vi "Actor Core.vi"(8 "error in":errorcluster, 11 "User Interface in":refnum<class "User Interface.lvclass">) -> (0 "error out":errorcluster, 3 "Actor out":refnum<class "Actor.lvclass">)   [LabVIEW 2022 SP3, in "User Interface.lvlib" / "User Interface.lvclass"]
doc: "(<B>Filename</B>: Actor Framework.lvlib:Actor.lvclass:Actor Core.vi)\n\nReceives messages to the actor, reacts to them, and initiates any error handling that may shut the actor down.\n\nDescendant classes may override this VI to append parallel tasks for the actor to complete while it handles messages. Overrides use the Call Parent Class Method node."
uses:
  User Interface.lvclass
  User Interface.lvclass/User Interface.ctl
  <vilib>/ActorFramework/Actor/Actor.lvclass
  Controls/UI States.ctl
  User Interface.lvlib
  <vilib>/ActorFramework/Stop Msg/Stop Msg.lvclass
  C:/Program Files/National Instruments/LabVIEW 2022/vi.lib/ActorFramework/Actor/Actor.lvclass
  E:/image-harvest/User Interface/User Interface/User Interface.lvclass
panel:
  in  "Settings":bool
  in  "Stop":bool
  in  "Start":bool
  out "Progress Bar":u8(slide) scale=0.0..100.0
  in  "Listbox":i32(listbox)
  out "Image":T1(plugin-control)
  # "Start"
  # "Stop"
  # "Settings"
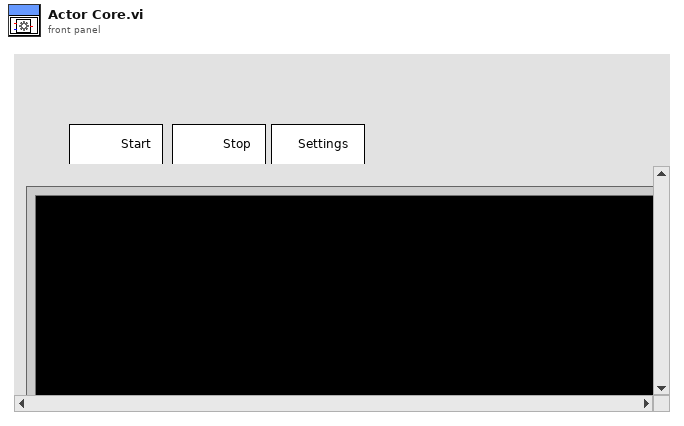
[diagram p1: front panel]
types:
  T1 = typedef "IMAQ Image.ctl" = refnum<image>
  T2 = typedef "User Interface.lvlib/UI States.ctl" = enum16{"Poll", "Initialize", "Start Acquisition", "Stop Acquisition", "Settings", "Error", "Exit"}
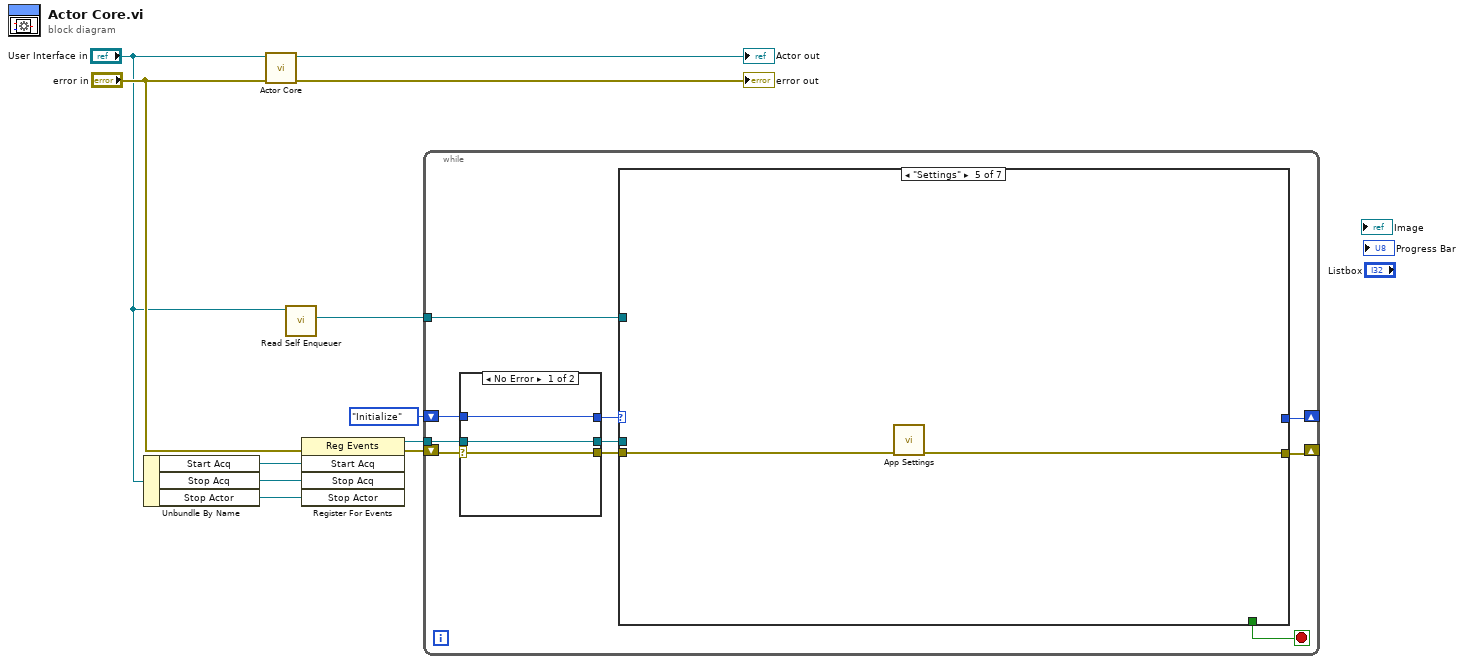
[diagram p0: block diagram]
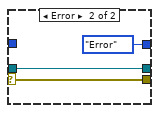
[diagram p2: hidden frame]
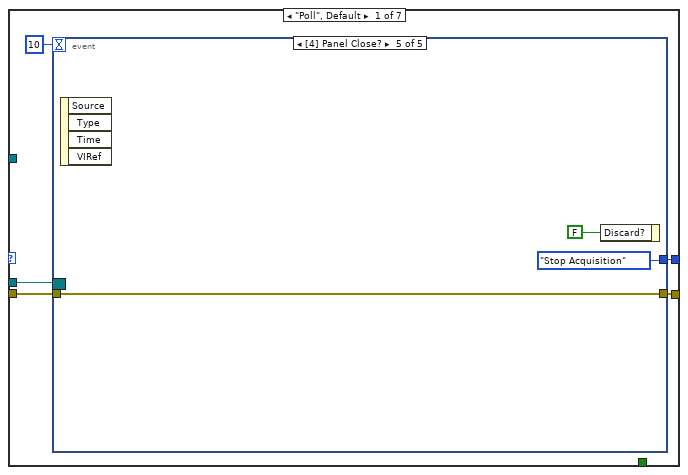
[diagram p3: hidden frame]
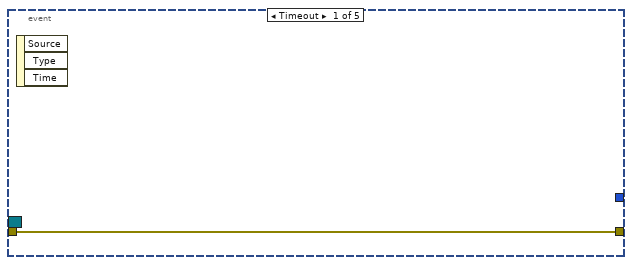
[diagram p4: hidden frame]
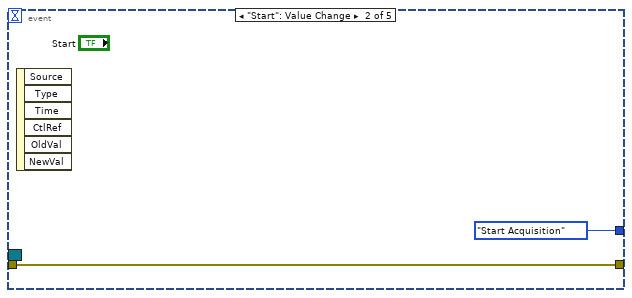
[diagram p5: hidden frame]
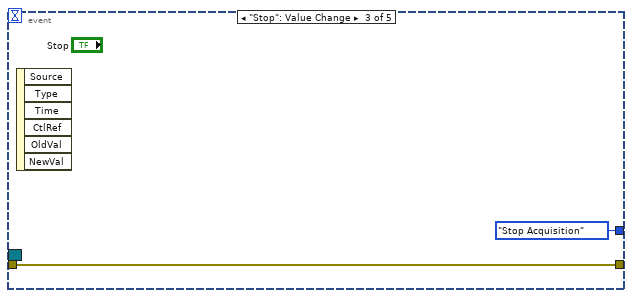
[diagram p6: hidden frame]
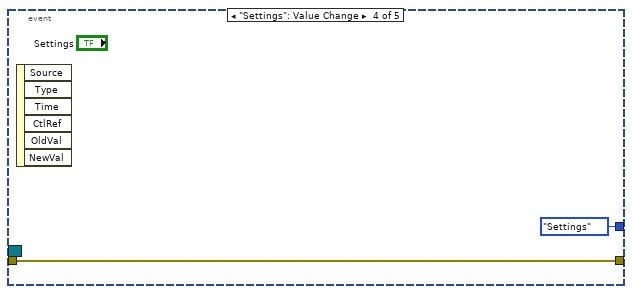
[diagram p7: hidden frame]
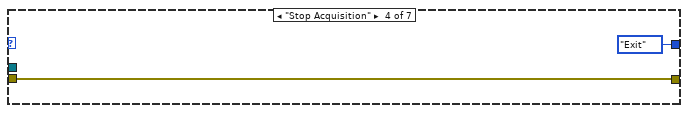
[diagram p10: hidden frame]
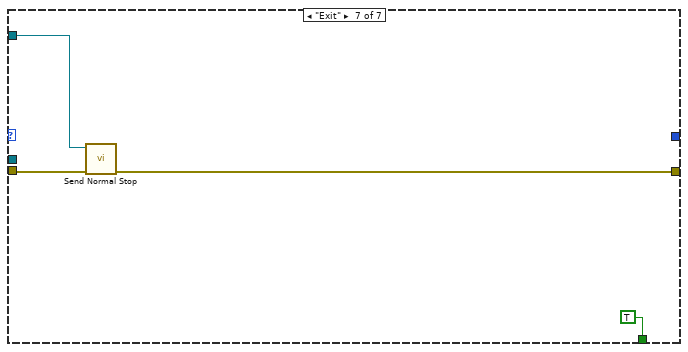
[diagram p12: hidden frame]
diagram:
  n1 = Unbundle By Name("User Interface in") -> ("Start Acq"=w8:refnum<user-event>, "Stop Acq"=w6:refnum<user-event>, "Stop Actor"=w7:refnum<user-event>)
  n2 = call-parent "Actor Core.vi"("error in"="error in", "Actor in"="User Interface in") -> ("error out"=→"error out":errorcluster, "Actor out"=→"Actor out":refnum<class "Actor.lvclass">)  [unwired: 8 in]
  n3 = call <vilib>:"Read Self Enqueuer.vi"("Actor"="User Interface in") -> ("Self Enqueuer"=w1:refnum<class "Message Enqueuer.lvclass">)  [unwired: 10 in]
  n4 = register-events(error in="error in", w8, w6, w7) -> (reference out=w4:refnum<event-registration>, error out=w3:errorcluster)  [unwired: 1 in]
  n5 = while {
    shift-right: [w21] -> _
    shift-left: UI_States."Initialize" -> [w18]
    tunnel: w4 -> [w17]
    shift-right: [w12] -> _
    shift-left: w3 -> [w20]
    tunnel: w1 -> [w13]
    stop <- w14 stop-if-true
    n6 = case shown="No Error" w20 {
      selector: w20 -> [w22 w26]
      tunnel: [w24 UI_States."Error"] -> w19
      tunnel: w18 -> [w24 _]
      tunnel: w17 -> [w23 w25]
      tunnel: [w23 w25] -> w16
      tunnel: [w22 w26] -> w15
      frame No Error {
      }
      frame Error {
      }
    }
    n7 = case shown="\"Settings\"" w19 {
      tunnel: w16 -> [w32 _ _ _ _ _ _]
      tunnel: [w31 _ _ UI_States."Exit" _ _ _] -> w21
      tunnel: w15 -> [w29 w43 w44 w46 w48 w49 w51]
      tunnel: [_ _ _ _ _ _ TRUE] -> w14
      tunnel: w13 -> [_ _ _ _ _ _ w52]
      tunnel: [w28 w43 w44 w46 w47 w49 w50] -> w12
      frame "Poll", Default {
        n8 = event shown="[4] Panel Close?" {
          selector: w32 -> [_ _ _ _ _]
          dyn-events: _ -> [_ _ _ _ _]
          timeout: 10 -> [_ _ _ _ _]
          tunnel: [_ UI_States."Start Acquisition" UI_States."Stop Acquisition" UI_States."Settings" UI_States."Stop Acquisition"] -> w31
          tunnel: w29 -> [w33 w34 w36 w38 w41]
          tunnel: [w33 w34 w36 w38 w41] -> w28
          event Timeout {
            n9 = event-data() -> ()  [unwired: 1 in, 3 out]
          }
          event "Start": Value Change {
            n10 = event-data() -> ()  [unwired: 1 in, 6 out]
          }
          event "Stop": Value Change {
            n11 = event-data() -> ()  [unwired: 1 in, 6 out]
          }
          event "Settings": Value Change {
            n12 = event-data() -> ()  [unwired: 1 in, 6 out]
          }
          event Panel Close? {
            n13 = event-data() -> ()  [unwired: 1 in, 4 out]
            n14 = event-data("Discard?"=FALSE) -> ()  [unwired: 1 in, 1 out]
          }
        }
      }
      frame "Initialize" {
      }
      frame "Start Acquisition" {
      }
      frame "Stop Acquisition" {
      }
      frame "Settings" {
        n15 = call "App Settings.vi"("Error in (no error)"=w48) -> ("Error out"=w47:errorcluster)  [unwired: 10 in]
      }
      frame "Error" {
      }
      frame "Exit" {
        n16 = call <vilib>:"Send Normal Stop.vi"("error in (no error)"=w51, "Message Enqueuer"=w52) -> ("error out"=w50:errorcluster)  [unwired: 9 in]
      }
    }
  }
